vi "CommandClient.vi"(4 "ms Wait Before Read":u32=50, 6 "sec Timeout":u32=500, 8 "error in":errorcluster, 10 "Command":string, 11 "Comport":refnum<visa-resource-name>="COM8") -> (0 "error out":errorcluster, 1 "Last Entry":string, 2 "Reply":string, 3 "Comport Out":refnum<visa-resource-name>)   [LabVIEW 2020, in "MicroPython.lvlib"]
doc: "Sends a command to a micropython target. The VI adds \"\\r\" to the message."
uses:
  MicroPython.lvlib
  <vilib>/regexp/Match Regular Expression.xnode
  SerialTxRx/SerialTxRx.lvlib
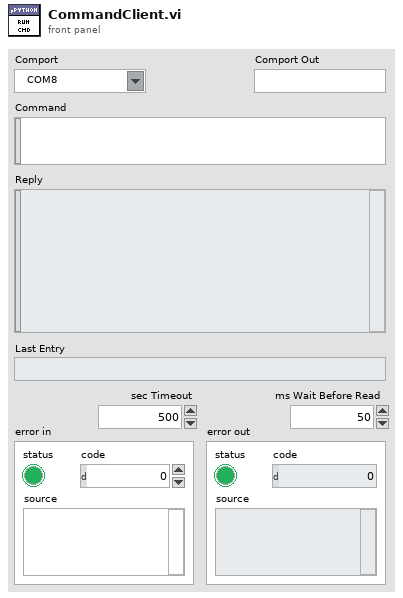
[diagram p1: front panel]
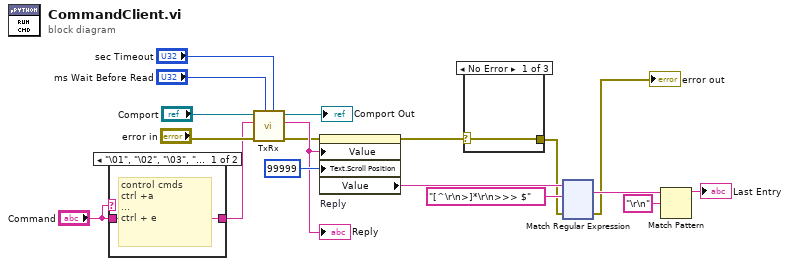
[diagram p0: block diagram]
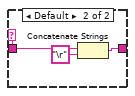
[diagram p2: hidden frame]
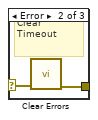
[diagram p3: hidden frame]
diagram:
  n1 = case shown="\"\\01\", \"\\02\", \"\\03\", \"\\04\", \"\\05\"" "Command" {
    selector: "Command" -> [_ w20]
    tunnel: "Command" -> [w19 _]
    tunnel: [w19 w21] -> w5
    frame "\u0001", "\u0002", "\u0003", "\u0004", "\u0005" {
      # "control cmds\nctrl +a\n...\nctrl + e"
    }
    frame Default {
      n2 = Concatenate Strings(w20, "\r" ("string")) -> (w21:string)
    }
  }
  n3 = call "TxRx.vi"("ms Timeout"="sec Timeout", "ms Wait Before Read"="ms Wait Before Read", "error in"="error in", "Tx Message"=w5, "VISA Resource Name In"="Comport") -> ("error out"=w2:errorcluster, "Rx Message"=w13:string, "VISA Resource Name Out"=→"Comport Out":refnum<visa-resource-name>)  [unwired: 4 in]
  "Reply" <- w13
  n4 = property on="Reply" class="Str"(error in=w2, "Value"=w13, "Text.Scroll Position"=u32 99999 ("byte count")) -> (error out=w1:errorcluster, "Value"=w7:string)  [unwired: 1 in, 1 out]
  n5 = case shown="No Error" w1 {
    selector: w1 -> [w23 w25 w26]
    tunnel: [w23 w24 w26] -> w4
    frame No Error {
    }
    frame Error {
      # "Clear Timeout"
      n6 = call <vilib>:"Clear Errors.vi"("error in (no error)"=w25) -> ("error out"=w24:errorcluster)  [unwired: 5 in, 1 out]
    }
    frame Default {
    }
  }
  n7 = xnode "Match Regular Expression"("input string"=w7, "regular expression"="[^\r\n>]*\r\n>>> $", "error in"=w4) -> ("whole match"=w17:string, "error out"=→"error out":errorcluster)  [unwired: 3 in, 3 out]
  n8 = Match Pattern(string=w17, regular expression="\r\n") -> (before substring=→"Last Entry":string)  [unwired: 1 in, 3 out]
